vi "numToHex_LE.vi"(1 "Numeric":sgl) -> (0 "string":string)   [LabVIEW 2015]
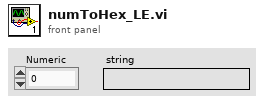
[diagram p1: front panel]
types:
  T1 = enum16{"big-endian, network order", "native, host order", "little-endian"}
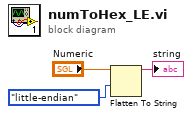
[diagram p0: block diagram]
diagram:
  n1 = Flatten To String(anything="Numeric", byte order (0:big-endian, network order)=T1."little-endian") -> (data string=→"string":string)  [unwired: 2 in, 2 out]
